vi "Get Picture.vi"(8 "error in (no error)":errorcluster, 11 "Chemicals in":refnum<class "Chemicals.lvclass">) -> (0 "error out":errorcluster, 2 "Picture":picture, 3 "Chemicals out":refnum<class "Chemicals.lvclass">)   [LabVIEW 2020, in "Chemicals.lvclass"]
uses:
  Chemicals.lvclass
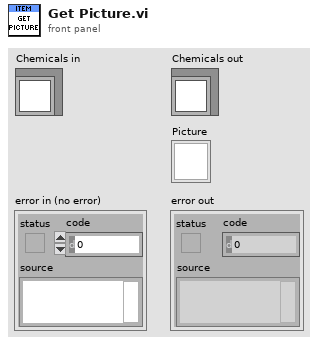
[diagram p1: front panel]
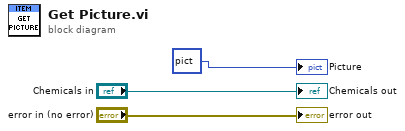
[diagram p0: block diagram]
diagram:
  "error out" <- "error in (no error)"
  "Chemicals out" <- "Chemicals in"
  "Picture" <- picture bytes[3230] ("new picture")
